vi "GFV DG Systems.vi"(0 "BME_DG_System":refnum<class "BME_DG_System.lvclass">, 5 "SystemlName":string, 7 "Config File":path, 9 "Dir Calibration files":path, 11 "error in":errorcluster, 12 "Mode":T1(ring)) -> (4 "BME_DG_System out":refnum<class "BME_DG_System.lvclass">, 6 "ChnlNames":string[](array[string]), 8 "Initialized?":bool, 10 "new Modules.cal?":bool, 14 "Problem Chnls out":string[](array[string]), 15 "error out":errorcluster)   [LabVIEW 2009, in "POLARIS BME DG.lvlib" / "BME_DG_System.lvclass"]
uses:
  BME_DG_System.lvclass
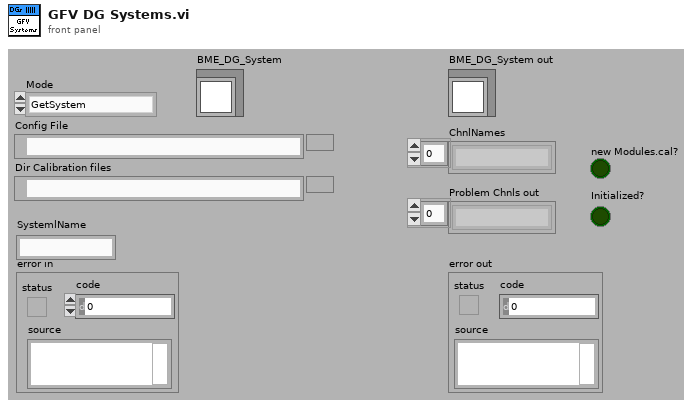
[diagram p1: front panel]
types:
  T1 = enum16{"GetSystem", "SetSystem", "FirstInit", "ForceInit", "Release"}
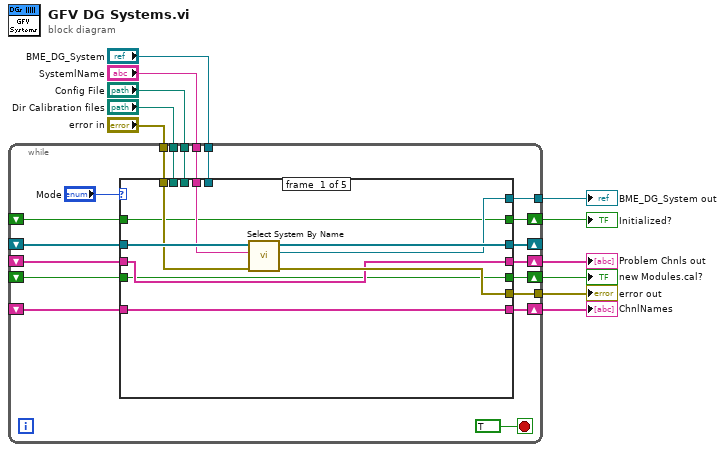
[diagram p0: block diagram]
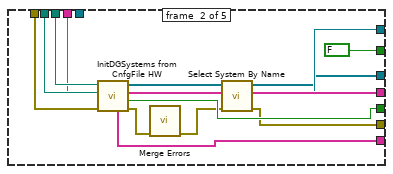
[diagram p2: hidden frame]
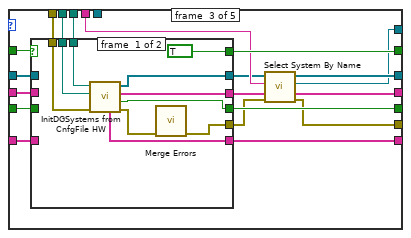
[diagram p3: hidden frame]
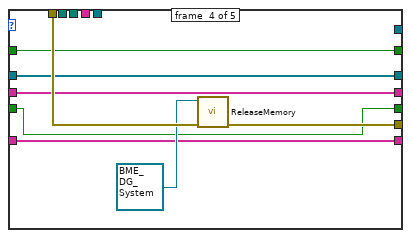
[diagram p5: hidden frame]
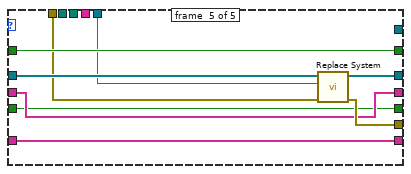
[diagram p6: hidden frame]
diagram:
  n1 = while {
    shift-right: [w28] -> _
    shift-left: _ -> [w20]
    shift-right: [w29] -> w10
    shift-left: _ -> [w19]
    shift-right: [w30] -> w11
    shift-left: _ -> [w18]
    tunnel: "Config File" -> [w25]
    tunnel: "Dir Calibration files" -> [w24]
    tunnel: "error in" -> [w23]
    shift-right: [w22] -> w5
    shift-left: _ -> [w21]
    shift-right: [w27] -> w9
    shift-left: _ -> [w17]
    tunnel: [w16] -> w4
    tunnel: "SystemlName" -> [w15]
    tunnel: [w14] -> w2
    tunnel: "BME_DG_System" -> [w13]
    stop <- TRUE stop-if-true
    n2 = case shown="\"FirstInit\"" "Mode" {
      tunnel: [w37 w43 w55 w95 w102] -> w16
      tunnel: [w32 w54 w67 w90 w98] -> w30
      tunnel: [w33 w53 w68 w91 w99] -> w29
      tunnel: [w39 w41 w58 w92 w103] -> w28
      tunnel: [w31 w52 w66 w89 w97] -> w27
      tunnel: w25 -> [_ w51 w71 _ _]
      tunnel: w24 -> [_ w50 w70 _ _]
      tunnel: w23 -> [w38 w49 w69 w96 w101]
      tunnel: [w34 FALSE w61 w93 w105] -> w22
      tunnel: w21 -> [w34 _ w72 w93 w105]
      tunnel: w20 -> [w40 _ w65 w92 w104]
      tunnel: w19 -> [w33 _ w64 w91 w99]
      tunnel: w18 -> [w32 _ w63 w90 w98]
      tunnel: w17 -> [w31 _ w62 w89 w97]
      tunnel: w15 -> [w36 w45 w60 _ _]
      tunnel: [w35 w42 w57 _ _] -> w14
      tunnel: w13 -> [_ _ _ _ w100]
      frame #0 {
        n3 = call "Select System By Name.vi"("error in (no error)"=w38, "SystemlName"=w36, "SystemsIn"=w40) -> ("error out"=w37:errorcluster, "BME_DG_System out"=w35:refnum<class "BME_DG_System.lvclass">, "SystemsOut"=w39:refnum<class "BME_DG_System.lvclass">[])  [unwired: 6 in]
      }
      frame #1 {
        n4 = call "InitDGSystems from CnfgFile HW.vi"("error in"=w49, "Dir Calibration files"=w50, "Config File"=w51) -> ("Errors"=w47:errorcluster[], "new Modules.cal?"=w54:bool, "Problem Chnls out"=w53:string[], "DG Systems"=w46:refnum<class "BME_DG_System.lvclass">[], "ChnlNames"=w52:string[])  [unwired: 4 in]
        n5 = call <vilib>:"Merge Errors.vi"("error array in"=w47) -> ("error out"=w44:errorcluster)  [unwired: 6 in]
        n6 = call "Select System By Name.vi"("error in (no error)"=w44, "SystemlName"=w45, "SystemsIn"=w46) -> ("error out"=w43:errorcluster, "BME_DG_System out"=w42:refnum<class "BME_DG_System.lvclass">, "SystemsOut"=w41:refnum<class "BME_DG_System.lvclass">[])  [unwired: 6 in]
      }
      frame #2 {
        n7 = case shown="False" w72 {
          selector: w72 -> [_ w83]
          tunnel: w71 -> [w82 _]
          tunnel: w70 -> [w81 _]
          tunnel: w69 -> [w80 w84]
          tunnel: [w74 w88] -> w59
          tunnel: [w79 w87] -> w68
          tunnel: [w78 w86] -> w67
          tunnel: [w73 w84] -> w56
          tunnel: [w77 w85] -> w66
          tunnel: w65 -> [_ w88]
          tunnel: w64 -> [_ w87]
          tunnel: w63 -> [_ w86]
          tunnel: w62 -> [_ w85]
          tunnel: [TRUE w83] -> w61
          frame #0 {
            n8 = call "InitDGSystems from CnfgFile HW.vi"("error in"=w80, "Dir Calibration files"=w81, "Config File"=w82) -> ("Errors"=w76:errorcluster[], "new Modules.cal?"=w78:bool, "Problem Chnls out"=w79:string[], "DG Systems"=w74:refnum<class "BME_DG_System.lvclass">[], "ChnlNames"=w77:string[])  [unwired: 4 in]
            n9 = call <vilib>:"Merge Errors.vi"("error array in"=w76) -> ("error out"=w73:errorcluster)  [unwired: 6 in]
          }
          frame #1 {
          }
        }
        n10 = call "Select System By Name.vi"("error in (no error)"=w56, "SystemlName"=w60, "SystemsIn"=w59) -> ("error out"=w55:errorcluster, "BME_DG_System out"=w57:refnum<class "BME_DG_System.lvclass">, "SystemsOut"=w58:refnum<class "BME_DG_System.lvclass">[])  [unwired: 6 in]
      }
      frame #3 {
        n11 = call-dynamic "ReleaseMemory.vi"("error in (no error)"=w96, "BME_DG_System in"=refnum<class "BME_DG_System.lvclass"> refnum) -> ("error out"=w95:errorcluster)  [unwired: 8 in, 1 out]
      }
      frame #4 {
        n12 = call "Replace System.vi"("error in (no error)"=w101, "BME_DG_System"=w100, "SystemsIn"=w104) -> ("error out"=w102:errorcluster, "SystemsOut"=w103:refnum<class "BME_DG_System.lvclass">[])  [unwired: 7 in]
      }
    }
  }
  "new Modules.cal?" <- w11
  "Problem Chnls out" <- w10
  "ChnlNames" <- w9
  "Initialized?" <- w5
  "error out" <- w4
  "BME_DG_System out" <- w2
